vi "randomNumber.vi"() -> ()   [LabVIEW 2018]
panel:
  out "stop":bool
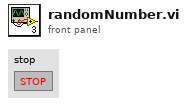
[diagram p1: front panel]
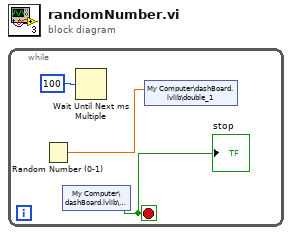
[diagram p0: block diagram]
diagram:
  n1 = while {
    stop <- w2 stop-if-true
    n2 = Random Number (0-1)() -> (number: 0 to 1=w1:dbl)
    n3 = shared-variable "My Computer\\dashBoard.lvlib\\stop"() -> (w2:bool)  [unwired: 1 in, 1 out]
    "stop" <- w2
    n4 = Wait Until Next ms Multiple(millisecond multiple=u32 100) -> ()  [unwired: 1 out]
    n5 = shared-variable "My Computer\\dashBoard.lvlib\\double_1"(w1) -> ()  [unwired: 1 in, 1 out]
  }
